vi "Read1000.vi"() -> ()   [LabVIEW 2015]
uses:
  <vilib>/Platform/TimedLoop/XDataNode/timing_clust.ctl
  <vilib>/Platform/TimedLoop/XDataNode/nitl_modes.ctl
  <vilib>/Platform/TimedLoop/XDataNode/wakeup.ctl
  <vilib>/platform/TimedLoop/XDataNode/XDataNode.xnode
  <vilib>/Platform/TimedLoop/XDataNode/XDNodeRunTimeDep.lvlib
panel:
  out "time":dbl
  out "x-y":i32
  out "appended array":i32[][][](array[numeric])
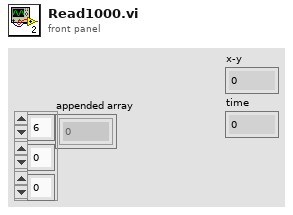
[diagram p1: front panel]
types:
  T1 = typedef "XDNodeRunTimeDep.lvlib/timing_clust.ctl" = cluster{"Expected End [f-1]":u64, "Actual End [f-1]":u64, "Finished Late? [f-1]":bool, "Expected End [i-1]":u64, "Actual End [i-1]":u64, "Finished Late? [i-1]":bool, "Expected Start [i]":u64, "Actual Start [i]":u64, "Expected Start [f]":u64, "Actual Start [f]":u64, "Source Name":string, "Structure Name":string, "Period":i64, "Deadline":i64, "Offset":i64, "Start":i64, "Priority":i32, "Timeout":i32, "Mode":T2, "Wakeup Reason":T3, "Error":errorcluster, "Source Type":string, "Secondary Source Type":string, "Global End Time":u64, "Global Start Time":u64, "Frame Duration":u64, "Iteration Duration":u64, "Assigned CPU":i32, "I/O Scan Engine Mode":u32}
  T2 = typedef "XDNodeRunTimeDep.lvlib/nitl_modes.ctl" = enum32{"No Change", "Process missed periods, maintain original phase", "Discard missed periods, maintain original phase", "Process missed periods, ignore original phase", "Discard missed periods, ignore original phase"}
  T3 = typedef "XDNodeRunTimeDep.lvlib/wakeup.ctl" = enum32{"Normal", "Aborted", "Asynchronous wakeup", "Timing source error", "Timed loop error", "Timeout"}
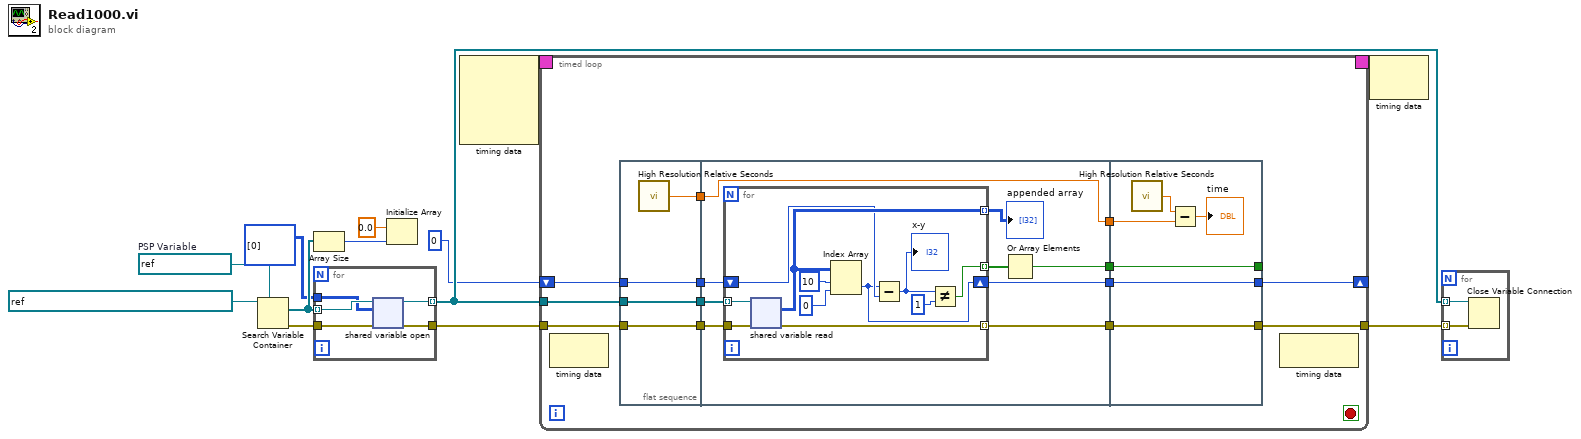
[diagram p0: block diagram]
diagram:
  w11 = refnum<k21> refnum  # PSP Variable
  n1 = Search Variable Container(7:w11, 11:refnum<k21> "ni.var.psp://my computer/Lib1000" ("container refnum in")) -> (0:w10:errorcluster, 2:w8:refnum<k21>[])  [unwired: 4 in, 1 out]
  n2 = Array Size(array=w8) -> (size(s)=w7:i32)
  n3 = for {
    tunnel: w8 -> [w18] mode=indexing
    tunnel: w10 -> [w17]
    tunnel: [w16] -> w4 mode=indexing
    tunnel: [w15] -> w9
    tunnel: i32[][] [[0]] ("appended array") -> [w14]
    n4 = shared-variable-open(w18, w17, w14) -> (w16:refnum<k21>, w15:errorcluster)  [unwired: 1 in]
  }
  n5 = Initialize Array(0.0 ("element"), w7) -> ()  [unwired: 1 out]
  n6 = node-c288() -> (w13:T1)  [unwired: 4 in]
  n7 = timed-loop {
    timing: w13 -> [_]
    timing-out: [_] -> w12
    tunnel: w4 -> [w31]
    tunnel: w9 -> [w30]
    tunnel: [w29] -> w5
    shift-right: [w27] -> _
    shift-left: 0 -> [w28]
    stop <- _ stop-if-true
    n8 = node-c288() -> ()  [unwired: 1 in, 1 out]
    n9 = flat-sequence {
      tunnel: w28 -> [w33]
      tunnel: w30 -> [w34]
      tunnel: w31 -> [w35]
      tunnel: [w35] -> w26
      tunnel: [w34] -> w25
      tunnel: [w33] -> w24
      tunnel: [w32] -> w20
      tunnel: w26 -> [w44]
      tunnel: w25 -> [w43]
      tunnel: w24 -> [w40]
      tunnel: [w42] -> w23
      tunnel: [w39] -> w22
      tunnel: [w38] -> w21
      tunnel: w20 -> [w38]
      tunnel: [w36] -> w19
      tunnel: [w60] -> w27
      tunnel: [w61] -> w29
      tunnel: w23 -> [w61]
      tunnel: w22 -> [w60]
      tunnel: w21 -> [w57]
      tunnel: [w56] -> _
      tunnel: w19 -> [w56]
      frame #0 {
        n10 = call <vilib>:"High Resolution Relative Seconds.vi"() -> ("relative seconds"=w32:dbl)
      }
      frame #1 {
        n11 = for {
          tunnel: w44 -> [w55] mode=indexing
          tunnel: w43 -> [w54]
          tunnel: [w53] -> w42 mode=indexing
          tunnel: [w52] -> w41 mode=indexing
          shift-right: [w45] -> w39
          shift-left: w40 -> [w51]
          tunnel: [w46] -> w37 mode=indexing
          n12 = shared-variable-read(w55, w54) -> (w53:errorcluster, w52:i32[][])  [unwired: 2 out]
          n13 = Index Array(array=w52, index (row)=10, index (col)=0 ("disabled index (col)")) -> (element=w45:i32)
          n14 = Subtract(x=w45, y=w51) -> (x-y=w48:i32)
          "x-y" <- w48
          n15 = Not Equal?(x=w48, y=1) -> (x != y?=w46:bool)
        }
        "appended array" <- w41
        n16 = Or Array Elements(Boolean array=w37) -> (logical OR=w36:bool)
      }
      frame #2 {
        n17 = call <vilib>:"High Resolution Relative Seconds.vi"() -> ("relative seconds"=w58:dbl)
        n18 = Subtract(x=w58, y=w57) -> (x-y=→"time":dbl)
      }
    }
    n19 = node-c288() -> ()  [unwired: 1 in, 1 out]
  }
  n20 = node-c288(w12) -> ()  [unwired: 1 out]
  n21 = for {
    tunnel: w5 -> [w65] mode=indexing
    tunnel: w4 -> [w64] mode=indexing
    n22 = Close Variable Connection(8:w65, 11:w64) -> ()  [unwired: 1 out]
  }
